vi "时间秒.vi"() -> (3 "结果字符串":string)   [LabVIEW 2020]
panel:
  in  "错误输入（无错误）":errorcluster
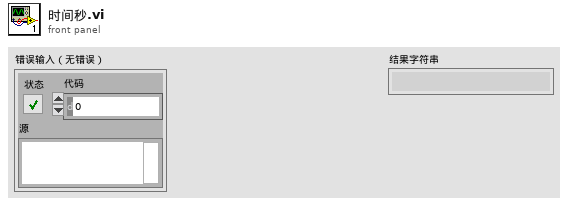
[diagram p1: front panel]
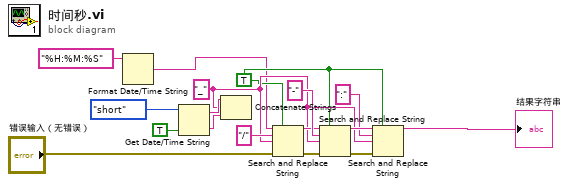
[diagram p0: block diagram]
diagram:
  w8 = TRUE ("替换全部？(F)")
  w9 = "_" ("替换字符串(\"\")")
  n1 = Format Date/Time String(time format string (%c)="%H:%M:%S" ("时间格式字符串(%c)")) -> (date/time string=w1:string)  [unwired: 2 in]
  n2 = Get Date/Time String(date format (0)=enum16{"short", "long", "abbreviated"}."short" ("日期格式(0)"), want seconds? (F)=TRUE ("需要秒？(F)")) -> (date string=w17:string, time string=w13:string)  [unwired: 1 in]
  n3 = Concatenate Strings(w17, w9, w13) -> ()  [unwired: 1 out]
  n4 = Search and Replace String(replace all?=w8, input string=w1, search string="/" ("搜索字符串"), replace string=w9, error in="错误输入（无错误）") -> (result string=w11:string, error out=w6:errorcluster)  [unwired: 3 in, 2 out]
  n5 = Search and Replace String(replace all?=w8, input string=w11, search string="-" ("搜索字符串"), replace string=w9, error in=w6) -> (result string=w15:string, error out=w5:errorcluster)  [unwired: 3 in, 2 out]
  n6 = Search and Replace String(replace all?=w8, input string=w15, search string=":" ("搜索字符串"), replace string=w9, error in=w5) -> (result string=→"结果字符串":string)  [unwired: 3 in, 3 out]
